vi "Deposit (SubVI).vi"(0 "Original balance":i32, 1 "database path":path, 2 "Deposit amount":i32, 3 "User row":i32, 4 "Array":string[][](array[string])) -> ()   [LabVIEW 2020]
uses:
  <vilib>/Utility/file.llb/Write Delimited Spreadsheet (string).vi
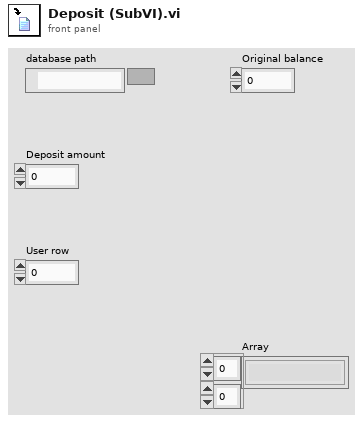
[diagram p1: front panel]
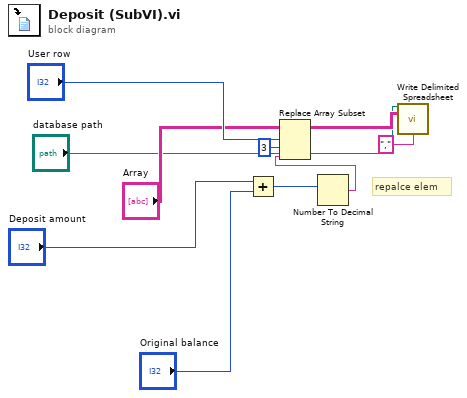
[diagram p0: block diagram]
diagram:
  # "repalce elem"
  n1 = Add(x="Deposit amount", y="Original balance") -> (x+y=w5:i32)
  n2 = Number To Decimal String(number=w5) -> (decimal integer string=w8:string)  [unwired: 1 in]
  n3 = Replace Array Subset "Replace Array Subset"(array="Array", new element=w8, index (row)="User row", index (col)=3 ("disabled index (col)")) -> (w6:string[][])
  n4 = call-poly <vilib>:"Write Delimited Spreadsheet.vi"("file path (dialog if empty)"="database path", "2D data"=w6, "delimiter (\\t)"="," ("delimiter (\\t)")) -> ()  [unwired: 11 in, 2 out]
